vi "ReadWrite TransConfig.vi"(7 "Mode":T1, 8 "error in (no error)":errorcluster, 11 "RT Data in":T2 {"Label Transfer Config"."Block Data Refs"."Data Reference" format="%.0x"; "Status Config"."HWOut Dur Ref" format="%.0x"; "Status Config"."HWIn Dur Ref" format="%.0x"; "Status Config"."Error Data Ref" format="%.0x"; "HWOutput Channels"."Labels Settings"."Label" format="%.0o"; "HWInput Channels"."Labels Settings"."Label" format="%.0o"}) -> (0 "error out":errorcluster, 3 "RT Data out":T2 {"Label Transfer Config"."Block Data Refs"."Data Reference" format="%.0x"; "Status Config"."HWOut Dur Ref" format="%.0x"; "Status Config"."HWIn Dur Ref" format="%.0x"; "Status Config"."Error Data Ref" format="%.0x"; "HWOutput Channels"."Labels Settings"."Label" format="%.0o"; "HWInput Channels"."Labels Settings"."Label" format="%.0o"})   [LabVIEW 2012, in "AIT 429 Engine.lvlib"]
uses:
  AIT 429 Engine.lvlib
  RT Controls/RT Data.ctl
  RT Controls/RT HW Channel.ctl
  RT Controls/RT Label Settings.ctl
  Shared/Controls and Global/Label.ctl
  Shared/Controls and Global/transferPeriod.ctl
  RT Controls/Driver Data.ctl
  RT Controls/RT Word Settings.ctl
  <vilib>/NI Veristand/Custom Device API/Block Data Reference.ctl
  <vilib>/NI Veristand/Custom Device API/Data Reference.ctl
  RT Controls/RT Param Setting.ctl
  Shared/Controls and Global/Start Bit.ctl
  Shared/Controls and Global/Number of Bits.ctl
  Shared/Controls and Global/TransferType.ctl
  RT Controls/Error Qs.ctl
  RT Controls/Status Channels Config.ctl
  RT Controls/FIFO.ctl
  RT Controls/Label Transfer Config.ctl
  RT Controls/ReadWrite Selector.ctl
  <vilib>/NI Veristand/Custom Device API/Global Data Refs.vi
  <vilib>/NI Veristand/Custom Device API/Custom Device API.lvlib
  ARINC 429 Shared.lvlib
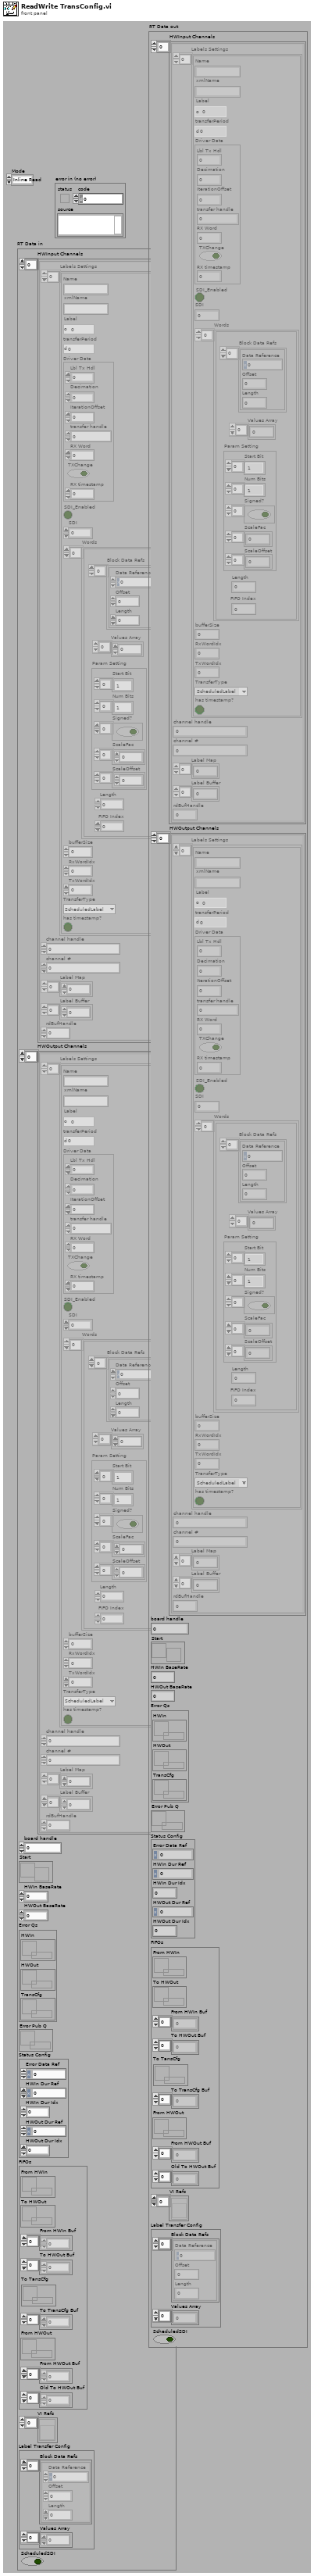
[diagram p1: front panel]
types:
  T1 = typedef "AIT 429 Engine.lvlib/ReadWrite Selector.ctl" = enum16{"Inline Read", "Inline Write", "Async HWIn", "Async HWOut"}
  T2 = typedef "AIT 429 Engine.lvlib/RT Data.ctl" = cluster{"HWInput Channels":T3[], "HWOutput Channels":T3[], "board handle":u32, "Start":refnum<notifier>, "HWIn BaseRate":i64, "HWOut BaseRate":i64, "Error Qs":T15, "Error Pub Q":refnum<queue>, "Status Config":T16, "FIFOs":T17, "VI Refs":refnum<vi>[], "Label Transfer Config":T18, "ScheduledSDI":bool}
  T3 = typedef "AIT 429 Engine.lvlib/RT HW Channel.ctl" = cluster{"Labels Settings":T4[], "channel handle":u32, "channel #":u16, "Label Map":i32[], "Label Buffer":u32[], "rdBufHandle":u32}
  T4 = typedef "AIT 429 Engine.lvlib/RT Label Settings.ctl" = cluster{"Name":string, "xmlName":string, "Label":T5, "transferPeriod":T6, "Driver Data":T7, "SDI_Enabled":bool, "SDI":u8, "Words":T8[], "bufferSize":u32, "RxWordIdx":i32, "TxWordIdx":i32, "TransferType":T14, "has timestamp?":bool}
  T5 = typedef "ARINC 429 Shared.lvlib/Label.ctl" = u8
  T6 = typedef "ARINC 429 Shared.lvlib/transferPeriod.ctl" = u32
  T7 = typedef "AIT 429 Engine.lvlib/Driver Data.ctl" = cluster{"Lbl Tx Hdl":u32, "Decimation":i32, "IterationOffset":i32, "transfer handle":u32, "RX Word":u32, "TXChange":bool, "RX timestamp":dbl}
  T8 = typedef "AIT 429 Engine.lvlib/RT Word Settings.ctl" = cluster{"Block Data Refs":T9[], "Values Array":dbl[], "Length":i32, "FIFO Index":i32, "Param Setting":T11}
  T9 = typedef "Custom Device API.lvlib/Block Data Reference.ctl" = cluster{"Data Reference":T10, "Offset":i32, "Length":i32}
  T10 = typedef "Custom Device API.lvlib/Data Reference.ctl" = i32
  T11 = typedef "AIT 429 Engine.lvlib/RT Param Setting.ctl" = cluster{"Start Bit":T12[], "Num Bits":T13[], "Signed?":bool[], "ScaleFac":dbl[], "ScaleOffset":dbl[]}
  T12 = typedef "ARINC 429 Shared.lvlib/Start Bit.ctl" = i32
  T13 = typedef "ARINC 429 Shared.lvlib/Number of Bits.ctl" = i32
  T14 = typedef "ARINC 429 Shared.lvlib/TransferType.ctl" = enum16{"ScheduledLabel", "Acyclic", "Block", "Strobe"}
  T15 = typedef "AIT 429 Engine.lvlib/Error Qs.ctl" = cluster{"HWIn":refnum<queue>, "HWOut":refnum<queue>, "TransCfg":refnum<queue>}
  T16 = typedef "AIT 429 Engine.lvlib/Status Channels Config.ctl" = cluster{"Error Data Ref":T10, "HWIn Dur Ref":T10, "HWIn Dur Idx":i32, "HWOut Dur Ref":T10, "HWOut Dur Idx":i32}
  T17 = typedef "AIT 429 Engine.lvlib/FIFO.ctl" = cluster{"From HWIn":refnum<k33>, "To HWOut":refnum<k33>, "From HWIn Buf":dbl[], "To HWOut Buf":dbl[], "To TansCfg":refnum<k33>, "To TransCfg Buf":dbl[], "From HWOut":refnum<k33>, "From HWOut Buf":dbl[], "Old To HWOut Buf":dbl[]}
  T18 = typedef "AIT 429 Engine.lvlib/Label Transfer Config.ctl" = cluster{"Block Data Refs":T9[], "Values Array":dbl[]}
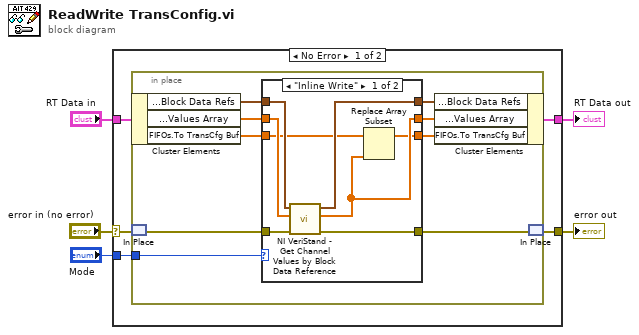
[diagram p0: block diagram]
diagram:
  n1 = case shown="No Error" "error in (no error)" {
    selector: "error in (no error)" -> [w9 w33]
    tunnel: "RT Data in" -> [w10 w32]
    tunnel: [w8 w32] -> w3
    tunnel: [w7 w33] -> w2
    tunnel: "Mode" -> [w6 _]
    frame No Error {
      n2 = in-place {
        in-place-border: w6 -> [w17]
        n3 = in-place-cluster #1(w10) -> ("Label Transfer Config.Block Data Refs"=w16:T9[], "Label Transfer Config.Values Array"=w15:dbl[], "FIFOs.To TransCfg Buf"=w12:dbl[])
        n4 = in-place-match #2(w9) -> (w19:errorcluster)
        n5 = case shown="\"Inline Write\"" w17 {
          tunnel: w19 -> [w26 w31]
          tunnel: [w23 w31] -> w18
          tunnel: w16 -> [w27 w30]
          tunnel: w15 -> [w25 w28]
          tunnel: [w21 w28] -> w14
          tunnel: [w24 w30] -> w13
          tunnel: w12 -> [w22 w29]
          tunnel: [w20 w29] -> w11
          frame "Inline Write" {
            n6 = call <vilib>:"NI VeriStand - Get Channel Values by Block Data Reference.vi"("error in (no error)"=w26, "Values Array in"=w25, "Block Data Ref"=w27) -> ("error out"=w23:errorcluster, "Values Array out"=w21:dbl[], "Block Data Ref dup"=w24:T9[])  [unwired: 6 in]
            n7 = Replace Array Subset(array=w22, new element=w21) -> (w20:dbl[])  [unwired: 1 in]
          }
          frame Default {
          }
        }
        n8 = in-place-cluster #1("Label Transfer Config.Block Data Refs"=w13, "Label Transfer Config.Values Array"=w14, "FIFOs.To TransCfg Buf"=w11) -> (w8:T2)
        n9 = in-place-match #2(w18) -> (w7:errorcluster)
      }
    }
    frame Error {
    }
  }
  "error out" <- w2
  "RT Data out" <- w3
